vi "step5 TestAndAlignUpperCross.vi"(11 "cube in":T1) -> (3 "cube out":T1)   [LabVIEW 2011]
uses:
  Typedef/cube.ctl
  Typedef/face.ctl
  Typedef/operation.ctl
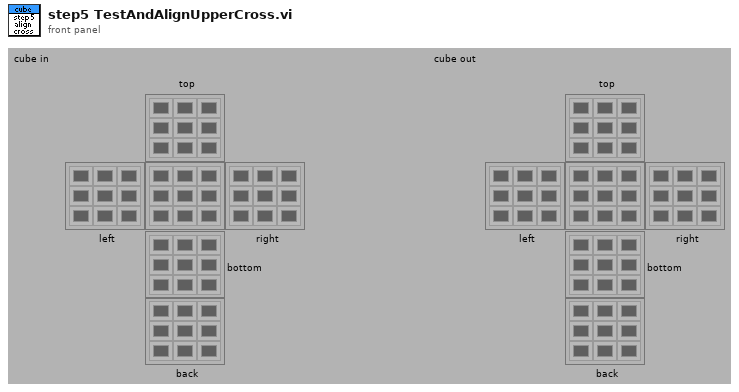
[diagram p1: front panel]
types:
  T1 = typedef "cube.ctl" = cluster{"top":T2, "left":T2, "right":T2, "bottom":T2, "back":T2, "front":T2}
  T2 = typedef "face.ctl" = u32[][]
  T3 = typedef "operation.ctl" = enum16{"nop", "T+", "T-", "F+", "F-", "L+", "L-", "R+", "R-", "B+", "B-", "<--", "-->", "^", "V"}
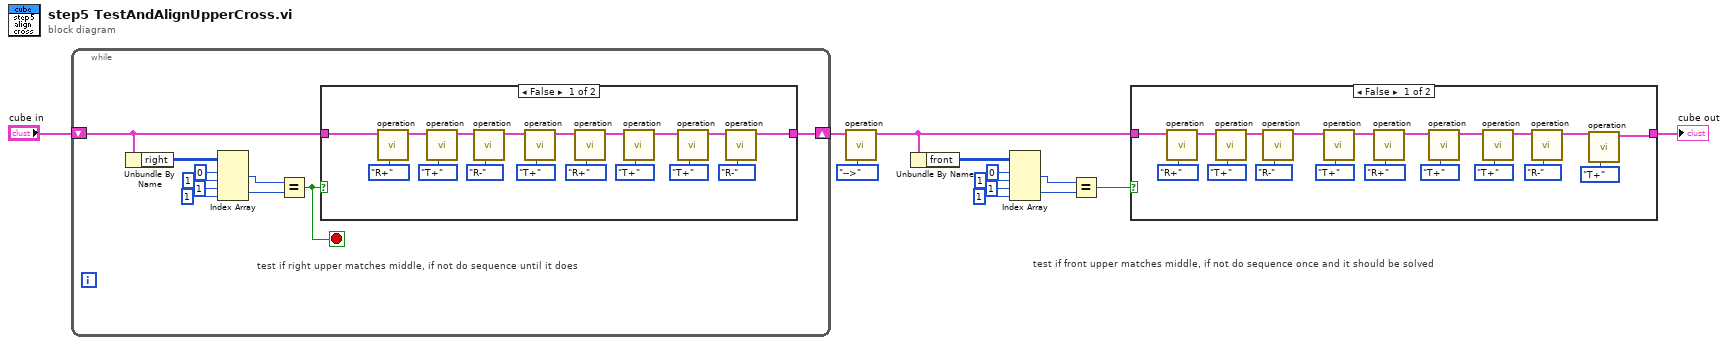
[diagram p0: block diagram]
diagram:
  # "test if front upper matches middle, if not do sequence once and it should be solved"
  n1 = while {
    shift-right: [w19] -> w2
    shift-left: "cube in" -> [w20]
    stop <- w14 stop-if-true
    # "test if right upper matches middle, if not do sequence until it does"
    n2 = Unbundle By Name(w20) -> ("right"=w21:T2)
    n3 = Index Array(array=w21, index (row) #1=0 ("index (row)"), index (col) #1=1 ("disabled index (col)"), index (row) #2=1 ("index (row)"), index (col) #2=1 ("disabled index (col)")) -> (element #1=w16:u32, element #2=w15:u32)
    n4 = Equal?(x=w16, y=w15) -> (x = y?=w14:bool)
    n5 = case shown="False" w14 {
      tunnel: w20 -> [w33 w41]
      tunnel: [w25 w41] -> w19
      frame False {
        n6 = call "operation.vi"("operation"=operation."R+", "cube in"=w33) -> ("cube out"=w32:T1)  [unwired: 8 in, 1 out]
        n7 = call "operation.vi"("operation"=operation."T+", "cube in"=w32) -> ("cube out"=w31:T1)  [unwired: 8 in, 1 out]
        n8 = call "operation.vi"("operation"=operation."R-", "cube in"=w31) -> ("cube out"=w30:T1)  [unwired: 8 in, 1 out]
        n9 = call "operation.vi"("operation"=operation."T+", "cube in"=w30) -> ("cube out"=w29:T1)  [unwired: 8 in, 1 out]
        n10 = call "operation.vi"("operation"=operation."R+", "cube in"=w29) -> ("cube out"=w28:T1)  [unwired: 8 in, 1 out]
        n11 = call "operation.vi"("operation"=operation."T+", "cube in"=w28) -> ("cube out"=w27:T1)  [unwired: 8 in, 1 out]
        n12 = call "operation.vi"("operation"=operation."T+", "cube in"=w27) -> ("cube out"=w26:T1)  [unwired: 8 in, 1 out]
        n13 = call "operation.vi"("operation"=operation."R-", "cube in"=w26) -> ("cube out"=w25:T1)  [unwired: 8 in, 1 out]
      }
      frame True {
      }
    }
  }
  n14 = call "operation.vi"("operation"=operation."-->", "cube in"=w2) -> ("cube out"=w1:T1)  [unwired: 8 in, 1 out]
  n15 = Unbundle By Name(w1) -> ("front"=w7:T2)
  n16 = Index Array(array=w7, index (row) #1=0 ("index (row)"), index (col) #1=1 ("disabled index (col)"), index (row) #2=1 ("index (row)"), index (col) #2=1 ("disabled index (col)")) -> (element #1=w10:u32, element #2=w11:u32)
  n17 = Equal?(x=w10, y=w11) -> (x = y?=w12:bool)
  n18 = case shown="False" w12 {
    tunnel: w1 -> [w43 w61]
    tunnel: [w42 w61] -> w4
    frame False {
      n19 = call "operation.vi"("operation"=operation."R+", "cube in"=w43) -> ("cube out"=w45:T1)  [unwired: 8 in, 1 out]
      n20 = call "operation.vi"("operation"=operation."T+", "cube in"=w45) -> ("cube out"=w44:T1)  [unwired: 8 in, 1 out]
      n21 = call "operation.vi"("operation"=operation."R-", "cube in"=w44) -> ("cube out"=w51:T1)  [unwired: 8 in, 1 out]
      n22 = call "operation.vi"("operation"=operation."T+", "cube in"=w51) -> ("cube out"=w52:T1)  [unwired: 8 in, 1 out]
      n23 = call "operation.vi"("operation"=operation."R+", "cube in"=w52) -> ("cube out"=w56:T1)  [unwired: 8 in, 1 out]
      n24 = call "operation.vi"("operation"=operation."T+", "cube in"=w56) -> ("cube out"=w53:T1)  [unwired: 8 in, 1 out]
      n25 = call "operation.vi"("operation"=operation."T+", "cube in"=w53) -> ("cube out"=w58:T1)  [unwired: 8 in, 1 out]
      n26 = call "operation.vi"("operation"=operation."R-", "cube in"=w58) -> ("cube out"=w60:T1)  [unwired: 8 in, 1 out]
      n27 = call "operation.vi"("operation"=operation."T+", "cube in"=w60) -> ("cube out"=w42:T1)  [unwired: 8 in, 1 out]
    }
    frame True {
    }
  }
  "cube out" <- w4
